vi "SecuenciaLEDS.vi"() -> ()   [LabVIEW 2020]
panel:
  in  "Stop Button":bool
  in  "Boolean":bool
  out "Array":bool[](array[boolean])
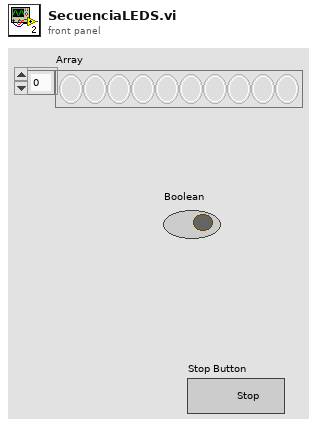
[diagram p1: front panel]
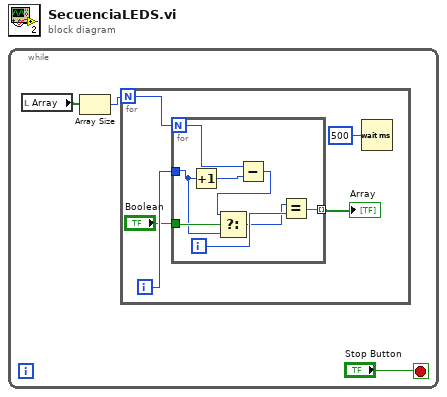
[diagram p0: block diagram]
diagram:
  n1 = while {
    stop <- "Stop Button" stop-if-true
    n2 = local read "Array"() -> (w2:bool[])
    n3 = Array Size(array=w2) -> (size(s)=w1:i32)
    n4 = for {
      N: w1 -> [w8]
      i -> [w7]
      n5 = for {
        N: w8 -> [w14]
        tunnel: w7 -> [w10]
        tunnel: [w15] -> w6 mode=indexing
        tunnel: "Boolean" -> [w12]
        i -> [w16]
        n6 = Increment(x=w10) -> (x+1=w13:i32)
        n7 = Subtract(x=w14, y=w13) -> (x-y=w11:i32)
        n8 = Select(t=w11, s=w12, f=w10) -> (s? t:f=w9:i32)
        n9 = Equal?(x=w9, y=w16) -> (x = y?=w15:bool)
      }
      "Array" <- w6
      n10 = Wait (ms)(milliseconds to wait=u32 500) -> ()  [unwired: 1 out]
    }
  }
